vi "read_exptime.vi"() -> ()   [LabVIEW 2015]
panel:
  out "comments":string[](array[string])
  out "lavgexp":i32
  out "error out":errorcluster caption="エラー出力"
  in  "error in":errorcluster caption="エラー入力"
  out "exp_sec":sgl
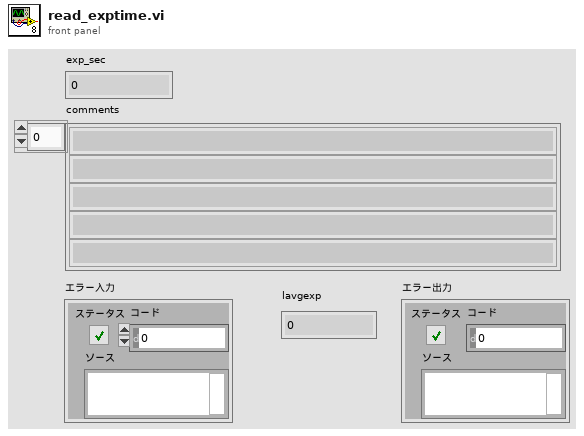
[diagram p1: front panel]
types:
  T1 = enum16{"open", "open or create", "create or replace", "create", "open (read only)"}
  T2 = enum16{"open", "replace", "create", "open or create", "replace or create", "replace or create with confirmation"}
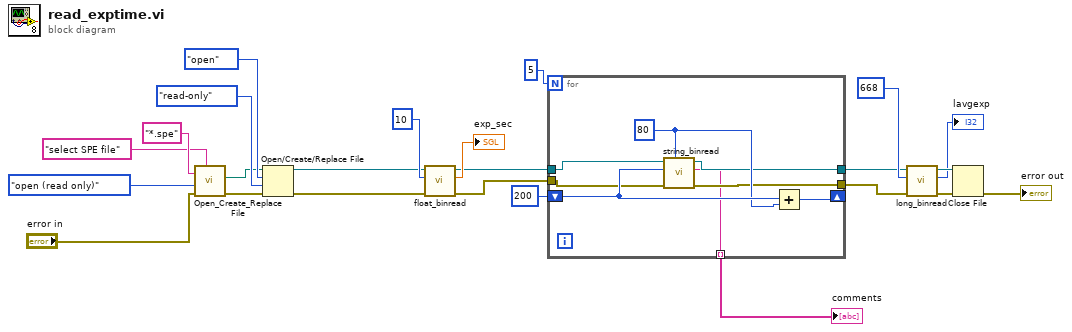
[diagram p0: block diagram]
diagram:
  n1 = call <vilib>:"Open_Create_Replace File.vi"("pattern"="*.spe", "prompt"="select SPE file", "error in (no error)"="error in", "function (open:0)"=T1."open (read only)") -> ("error out"=w20:errorcluster, "new file path"=w21:path)  [unwired: 4 in, 2 out]
  n2 = Open/Create/Replace File(file path (use dialog)=w21, error in=w20, operation (0:open)=T2."open", access (0:read/write)=enum16{"read/write", "read-only", "write-only"}."read-only" ("アクセス （0:read/write）")) -> (refnum out=w9:refnum<file>, error out=w8:errorcluster)  [unwired: 2 in, 1 out]
  n3 = call "float_binread.vi"("error in"=w8, "offset"=i64 10, "ref in"=w9) -> ("error out"=w4:errorcluster, "float"=→"exp_sec":sgl, "ref out"=w5:refnum<file>)  [unwired: 6 in]
  n4 = for {
    N: 5 -> [_]
    shift-right: [w32] -> _
    shift-left: 200 -> [w31]
    tunnel: w5 -> [w29]
    tunnel: w4 -> [w28]
    tunnel: [w27] -> w3
    tunnel: [w26] -> w2
    tunnel: [w25] -> w1 mode=indexing
    w30 = 80 ("length")
    n5 = call "string_binread.vi"("length"=w30, "error in"=w28, "offset"=w31, "ref in"=w29) -> ("error out"=w26:errorcluster, "string"=w25:string, "ref out"=w27:refnum<file>)  [unwired: 5 in]
    n6 = Add(x=w31, y=w30) -> (x+y=w32:i32)
  }
  "comments" <- w1
  n7 = call "long_binread.vi"("error in"=w2, "offset"=i64 668, "ref in"=w3) -> ("error out"=w15:errorcluster, "long"=→"lavgexp":i32, "ref out"=w14:refnum<file>)  [unwired: 6 in]
  n8 = Close File(refnum=w14, error in=w15) -> (error out=→"error out":errorcluster)  [unwired: 1 out]
